vi "Is Number a Date Cell.vi"(8 "error in":errorcluster, 10 "StyleIndex":refnum<k24>, 11 "SpreadsheetDoc in":refnum<k24>) -> (0 "error out":errorcluster, 1 "Is Date":bool, 2 "StyleIndex out":refnum<k24>, 3 "SpreadsheetDoc out":refnum<k24>)   [LabVIEW 2021, in "Open Xml.lvlib"]
uses:
  Open Xml.lvlib
  D:/git/Open-Xml-LabVIEW/dll/DocumentFormat.OpenXml.dll
  dll/DocumentFormat.OpenXml.dll
  D:/git/Open-Xml-LabVIEW/dll/DocumentFormat.OpenXml.Framework.dll
  dll/DocumentFormat.OpenXml.Framework.dll
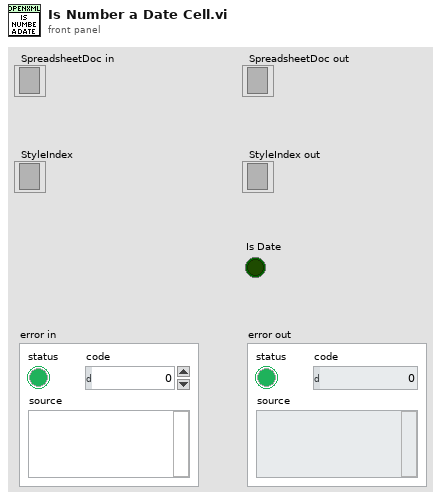
[diagram p1: front panel]
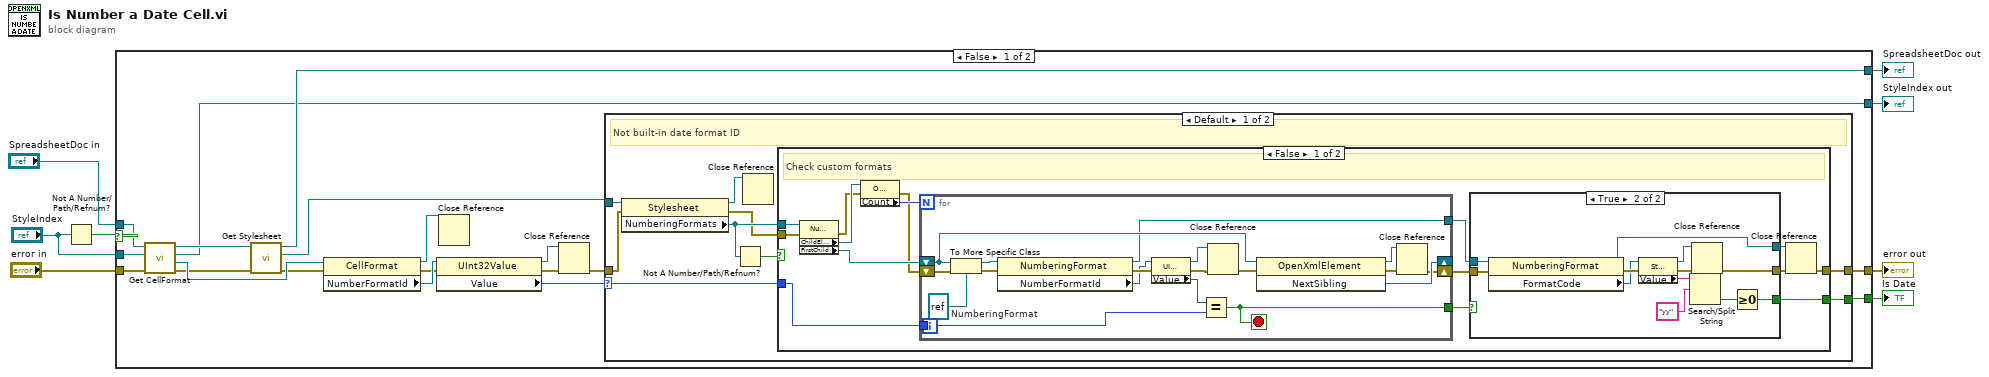
[diagram p0: block diagram]
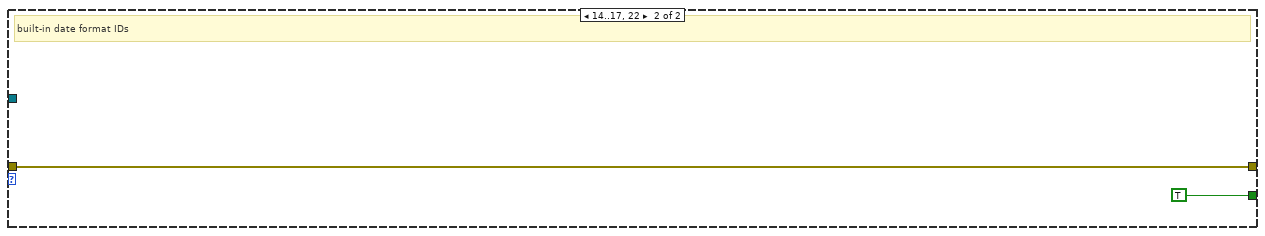
[diagram p4: hidden frame]
diagram:
  n1 = Not A Number/Path/Refnum?(number/path/refnum="StyleIndex") -> (NaN/Path/Refnum?=w6:bool)
  n2 = case shown="False" w6 {
    tunnel: "error in" -> [w26 w88]
    tunnel: [w22 _] -> w7
    tunnel: "StyleIndex" -> [w15 w87]
    tunnel: "SpreadsheetDoc in" -> [w27 w89]
    tunnel: [w12 w89] -> w4
    tunnel: [w16 w88] -> w3
    tunnel: [w9 w87] -> w1
    frame False {
      n3 = call "Get CellFormat.vi"("error in"=w26, "StyleIndex In"=w15, "SpreadsheetDocument in"=w27) -> ("error out"=w10:errorcluster, "CellFormat"=w25:refnum<k24>, "StyleIndex out"=w9:refnum<k24>, "SpreadsheetDocument out"=w13:refnum<k24>)  [unwired: 5 in]
      n4 = call "Get Stylesheet.vi"("error in"=w10, "SpreadsheetDoc in"=w13) -> ("error out"=w14:errorcluster, "Stylesheet"=w11:refnum<k24>, "SpreadsheetDoc out"=w12:refnum<k24>)  [unwired: 7 in]
      n5 = property class="CellFormat"(reference=w25, error in=w14) -> (reference out=w18:refnum<k24>, error out=w21:errorcluster, "NumberFormatId"=w24:refnum<k24>)
      n6 = property class="UInt32Value"(reference=w24, error in=w21) -> (reference out=w19:refnum<k24>, error out=w17:errorcluster, "Value"=w23:u32)
      n7 = Close Reference(reference=w18) -> ()  [unwired: 1 in, 1 out]
      n8 = Close Reference(reference=w19, error in (no error)=w17) -> (error out=w20:errorcluster)
      n9 = case shown="Default" w23 {
        selector: w23 -> [w32 _]
        tunnel: [w34 TRUE] -> w22
        tunnel: w20 -> [w28 w85]
        tunnel: w11 -> [w36 _]
        tunnel: [w31 w85] -> w16
        frame Default {
          # "Not built-in date format ID"
          n10 = property class="Stylesheet"(reference=w36, error in=w28) -> (reference out=w29:refnum<k24>, error out=w30:errorcluster, "NumberingFormats"=w33:refnum<k24>)
          n11 = Not A Number/Path/Refnum?(number/path/refnum=w33) -> (NaN/Path/Refnum?=w35:bool)
          n12 = Close Reference(reference=w29) -> ()  [unwired: 1 in, 1 out]
          n13 = case shown="False" w35 {
            tunnel: [w43 _] -> w34
            tunnel: w33 -> [w51 _]
            tunnel: w32 -> [w45 _]
            tunnel: [w38 w84] -> w31
            tunnel: w30 -> [w39 w84]
            frame False {
              # "Check custom formats"
              n14 = property class="NumberingFormats"(reference=w51, error in=w39) -> (error out=w48:errorcluster, "ChildElements"=w50:refnum<k24>, "FirstChild"=w47:refnum<k24>)  [unwired: 1 out]
              n15 = property class="OpenXmlElementList"(reference=w50, error in=w48) -> (error out=w46:errorcluster, "Count"=w49:i32)  [unwired: 1 out]
              n16 = for {
                N: w49 -> [_]
                shift-right: [w55] -> _
                shift-left: w47 -> [w58]
                shift-right: [w52] -> w41
                shift-left: w46 -> [w68]
                tunnel: w45 -> [w62]
                tunnel: [w57] -> w44
                tunnel: [w56] -> w40
                stop <- w56 stop-if-true
                w69 = refnum<k24> refnum  # NumberingFormat
                n17 = To More Specific Class(target class=w69, reference=w58, error in=w68) -> (specific class reference=w67:refnum<k24>, error out=w66:errorcluster)
                n18 = property class="NumberingFormat"(reference=w67, error in=w66) -> (reference out=w57:refnum<k24>, error out=w65:errorcluster, "NumberFormatId"=w64:refnum<k24>)
                n19 = property class="UInt32Value"(reference=w64, error in=w65) -> (reference out=w61:refnum<k24>, error out=w60:errorcluster, "Value"=w63:u32)
                n20 = Equal?(x=w63, y=w62) -> (x = y?=w56:bool)
                n21 = Close Reference(reference=w61, error in (no error)=w60) -> (error out=w59:errorcluster)
                n22 = invoke class="OpenXmlElement" method="NextSibling"(reference=w58, error in=w59) -> (reference out=w54:refnum<k24>, error out=w53:errorcluster, "NextSibling"=w55:refnum<k24>)  [unwired: 1 in]
                n23 = Close Reference(reference=w54, error in (no error)=w53) -> (error out=w52:errorcluster)
              }
              n24 = case shown="True" w40 {
                tunnel: w44 -> [w70 w83]
                tunnel: [_ w77] -> w43
                tunnel: [w71 w73] -> w42
                tunnel: w41 -> [w71 w75]
                tunnel: [w70 w72] -> w37
                frame False {
                }
                frame True {
                  n25 = property class="NumberingFormat"(reference=w83, error in=w75) -> (reference out=w72:refnum<k24>, error out=w82:errorcluster, "FormatCode"=w81:refnum<k24>)
                  n26 = property class="StringValue"(reference=w81, error in=w82) -> (reference out=w74:refnum<k24>, error out=w76:errorcluster, "Value"=w80:string)
                  n27 = Search/Split String(string=w80, search string/char (-)="yy") -> (offset of match=w78:i32)  [unwired: 1 in, 2 out]
                  n28 = Close Reference(reference=w74, error in (no error)=w76) -> (error out=w73:errorcluster)
                  n29 = Greater Or Equal To 0?(x=w78) -> (x >= 0?=w77:bool)
                }
              }
              n30 = Close Reference(reference=w37, error in (no error)=w42) -> (error out=w38:errorcluster)
            }
            frame True {
            }
          }
        }
        frame 14..17, 22 {
          # "built-in date format IDs"
        }
      }
    }
    frame True {
    }
  }
  "error out" <- w3
  "Is Date" <- w7
  "SpreadsheetDoc out" <- w4
  "StyleIndex out" <- w1
